vi "血压测试系统.vi"() -> ()   [LabVIEW 2014]
panel:
  out "血压计显示":dbl(slide) scale=0.0..120.0
  in  "血压计输入":dbl(slide) scale=0.0..120.0
  # "血压测试系统"
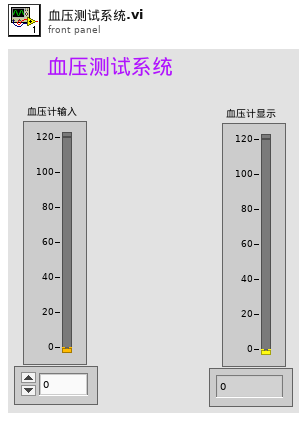
[diagram p1: front panel]
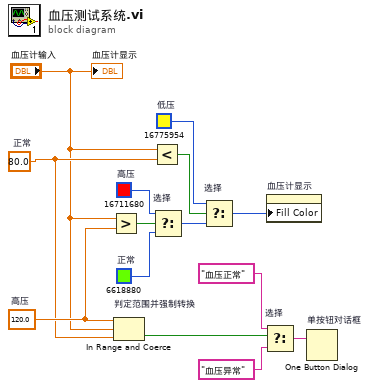
[diagram p0: block diagram]
diagram:
  w13 = u32 6618880  # 正常
  w10 = u32 16775954  # 低压
  w14 = u32 16711680  # 高压
  w4 = 120.0  # 高压
  w3 = 80.0  # 正常
  n1 = Greater?(x="血压计输入", y=w4) -> (0:w6:bool)
  n2 = In Range and Coerce "判定范围并强制转换"(upper limit=w4, x="血压计输入", lower limit=w3) -> (In Range?=w1:bool)  [unwired: 1 out]
  n3 = Less?(x="血压计输入", y=w3) -> (x < y?=w5:bool)
  n4 = Select "选择"(t=w14, s=w6, f=w13) -> (s? t:f=w11:u32)
  n5 = Select "选择"(t=w10, s=w5, f=w11) -> (s? t:f=w12:u32)
  n6 = Select "选择"(t="血压正常", s=w1, f="血压异常") -> (s? t:f=w7:string)
  n7 = property on="血压计显示" class="Slide (严格)"("Fill Color"=w12) -> ()  [unwired: 2 in, 2 out]
  n8 = One Button Dialog "单按钮对话框"(message=w7) -> ()  [unwired: 1 in, 1 out]
  "血压计显示" <- "血压计输入"
